vi "SubVI_Manipulador6DOF.vi"() -> (0 "error out":errorcluster, 3 "NI_Robotics_Serial Robot Arm out":refnum<class "NI_Robotics_Serial Robot Arm.lvclass">)   [LabVIEW 2017]
uses:
  <vilib>/robotics/Kinematics/Robot/NI_Robotics_Serial Robot Arm.lvclass
  <vilib>/robotics/Kinematics/Link/Joint Type.ctl
  <vilib>/robotics/Kinematics/Analytical/Initialize Generic Serial Arm.vi
  <vilib>/robotics/Kinematics/Link/NI_Robotics_Link.lvclass
  <vilib>/robotics/Kinematics/Analytical/NI_Robotics_AnalyticKinematics.lvlib
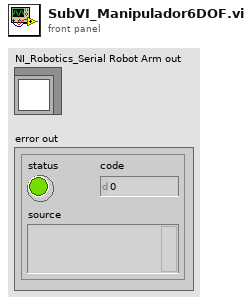
[diagram p1: front panel]
types:
  T1 = typedef "NI_Robotics_Link.lvclass/Joint Type.ctl" = enum16{"Revolute", "Prismatic"}
  T2 = cluster{"Twist Angle":dbl, "Length":dbl, "Rotation Angle":dbl, "Offset Distance":dbl, "Joint Type":T1, "Joint Coordinate Offset":dbl}[]
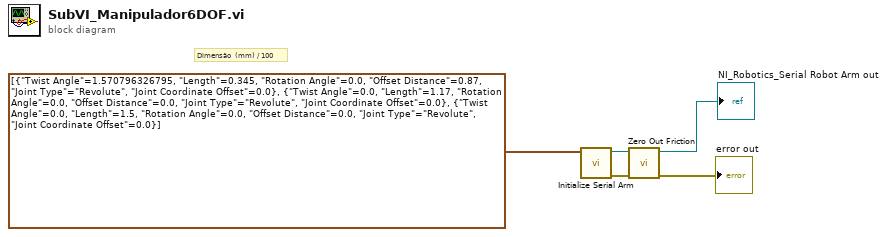
[diagram p0: block diagram]
diagram:
  # "Dimensão  (mm) / 100"
  n1 = call-poly <vilib>:"Initialize Serial Arm.vi"("kinematic parameters"=T2 [{"Twist Angle"=1.570796326795, "Length"=0.345, "Rotation Angle"=0.0, "Offset Distance"=0.87, "Joint Type"=enum."Revolute", "Joint Coordinate Offset"=0.0}, {"Twist Angle"=0.0, "Length"=1.17, "Rotation Angle"=0.0, "Offset Distance"=0.0, "Joint Type"=enum."Revolute", "Joint Coordinate Offset"=0.0}, {"Twist Angle"=0.0, "Length"=1.5, "Rotation Angle"=0.0, "Offset Distance"=0.0, "Joint Type"=enum."Revolute", "Joint Coordinate Offset"=0.0}]) -> ("error out"=w4:errorcluster, "serial arm out"=w3:refnum<class "NI_Robotics_Serial Robot Arm.lvclass">)  [unwired: 9 in]
  n2 = call <vilib>:"Zero Out Friction.vi"("error in (no error)"=w4, "serial arm in"=w3) -> ("error out"=→"error out":errorcluster, "serial arm out"=→"NI_Robotics_Serial Robot Arm out":refnum<class "NI_Robotics_Serial Robot Arm.lvclass">)  [unwired: 8 in]
